vi "Main.vi"(11 "Error In":errorcluster) -> (15 "Error Out":errorcluster)   [LabVIEW 2020]
doc: "The VI is a launcher VI that allows to perform the sender to receiver communication"
uses:
  Controls/Queue Operation.ctl
  Controls/User Event Operations.ctl
  Controls/Launcher Data.ctl
  Classes/Sender/Methods/Sender UI.vi
  Classes/Sender/Sender.lvclass
  Classes/Receiver/Methods/Receiver UI.vi
  Classes/Receiver/Receiver.lvclass
panel:
  # "Instructions:\n1. Run the VI.\n2. View the sender and receiver loaded in the front panel.\n3. Select the transmission data type.\n4. Click the notify button to send notification to the receiver.\n5. Click notify with data to send one data at a time.\n6. Click stream data to continuously stream data to the receiver and click stop stream to stop.\n7. Click panel close to stop the VI running"
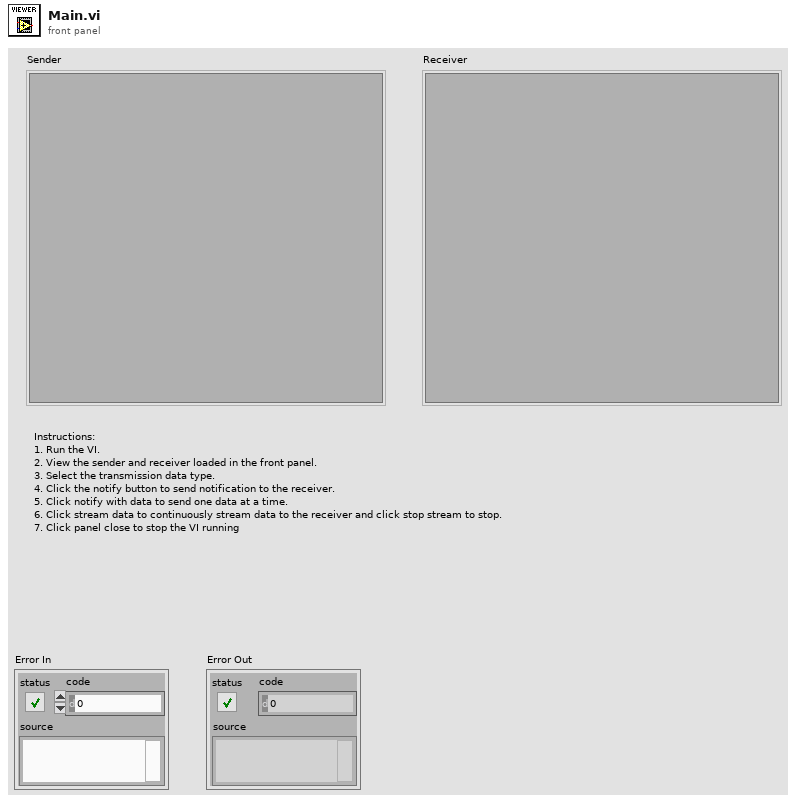
[diagram p1: front panel]
types:
  T1 = typedef "Launcher Data.ctl" = cluster{"Sender Reference":refnum<vi>, "Receiver Reference":refnum<vi>}
  T2 = typedef "User Event Operations.ctl" = enum16{"Obtain", "Generate", "Destroy"}
  T3 = typedef "Queue Operation.ctl" = enum16{"Create & Enqueue N", "Enqueue N", "Dequeue", "Enstack N", "Flush", "Release"}
  T4 = typedef "Queue Element.ctl" = cluster{"State":string, "Data":variant}
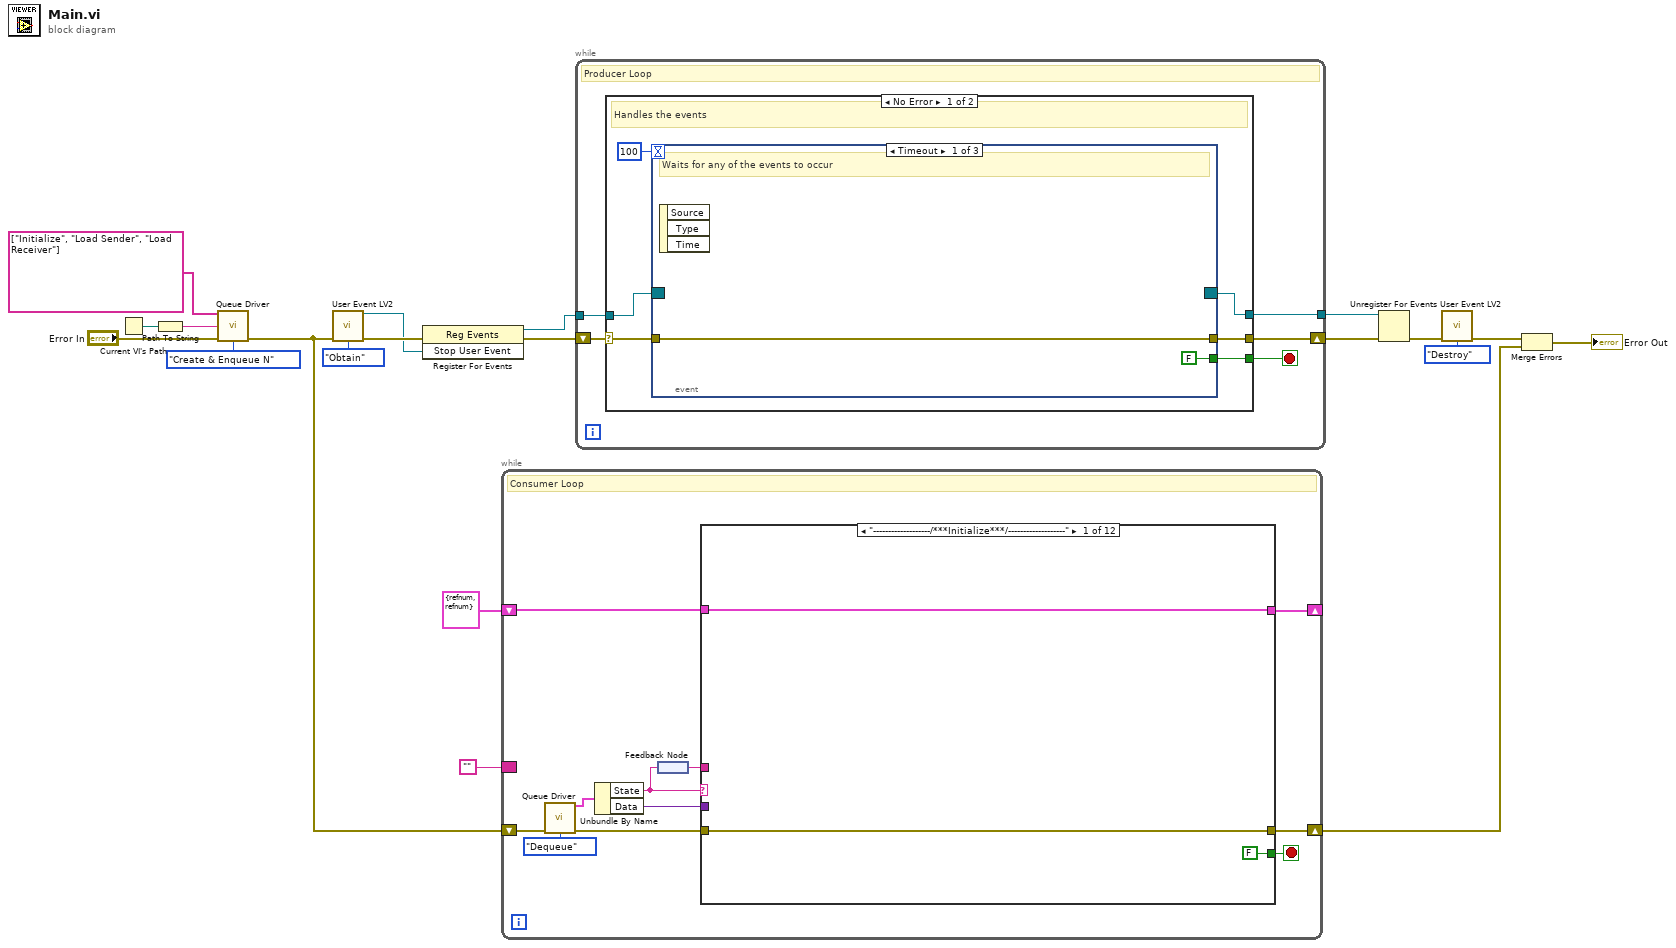
[diagram p0: block diagram]
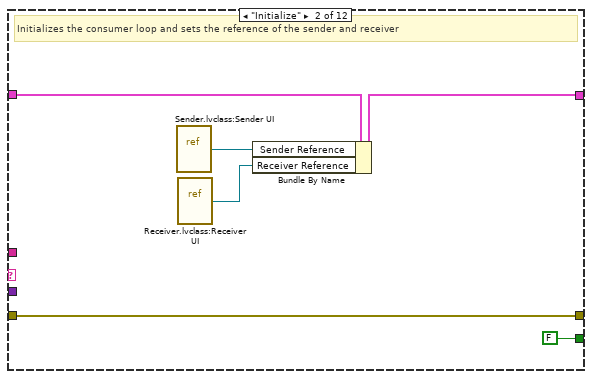
[diagram p2: hidden frame]
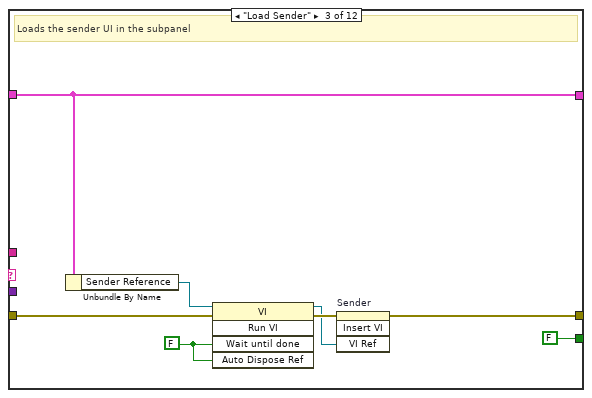
[diagram p3: hidden frame]
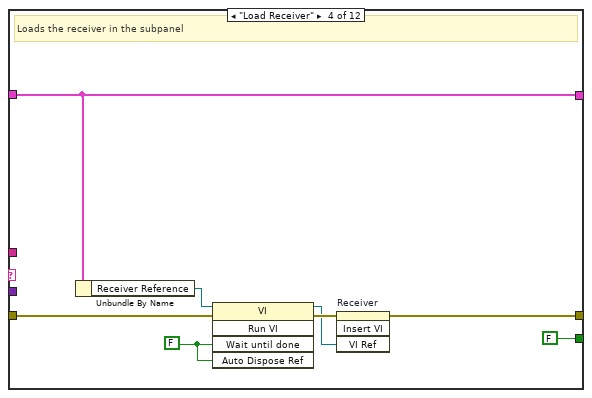
[diagram p4: hidden frame]
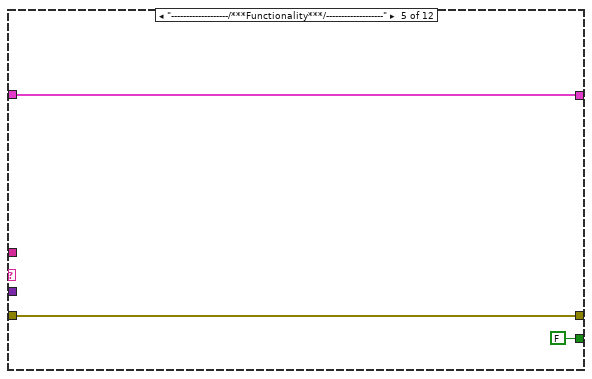
[diagram p5: hidden frame]
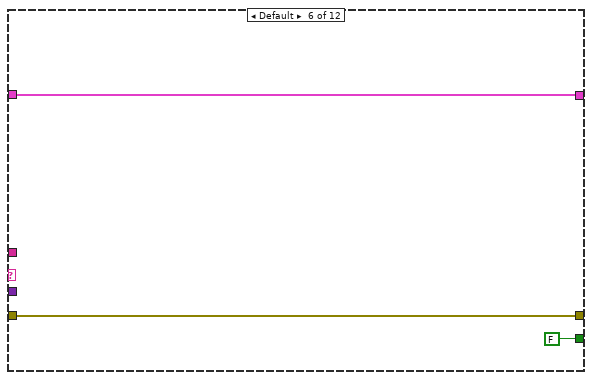
[diagram p6: hidden frame]
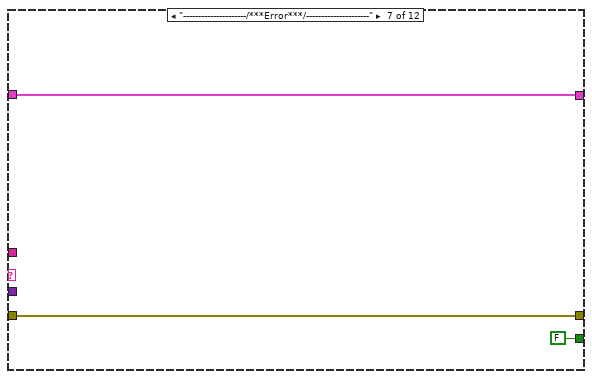
[diagram p7: hidden frame]
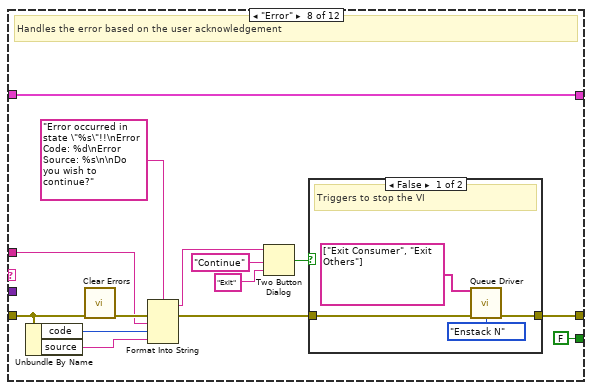
[diagram p8: hidden frame]
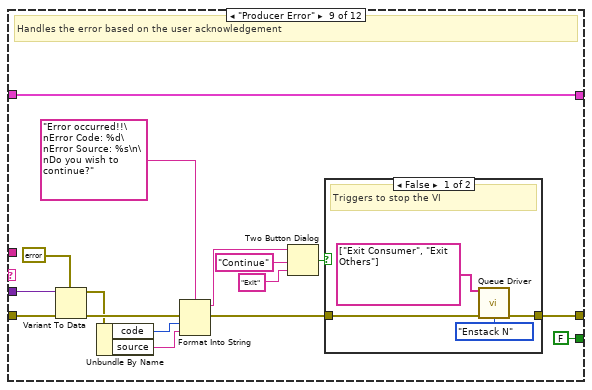
[diagram p10: hidden frame]
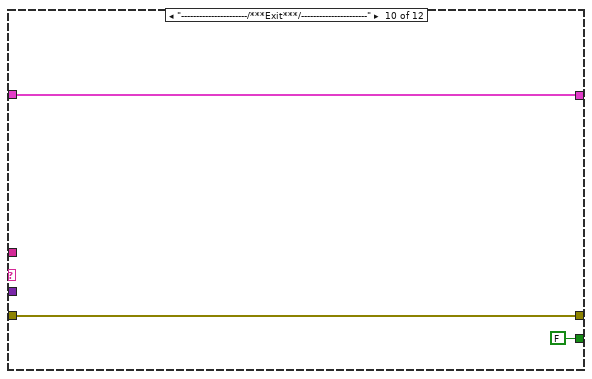
[diagram p12: hidden frame]
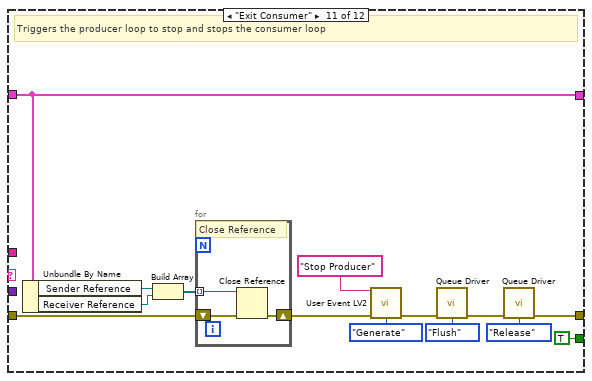
[diagram p13: hidden frame]
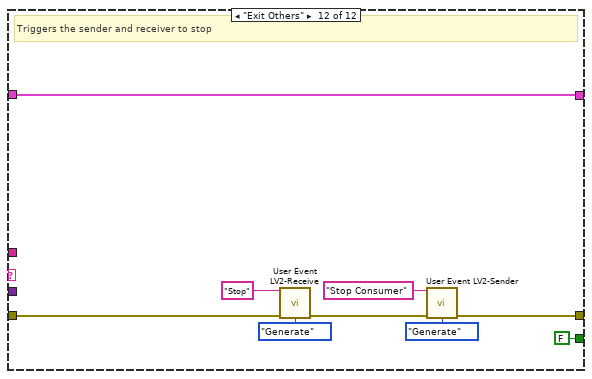
[diagram p14: hidden frame]
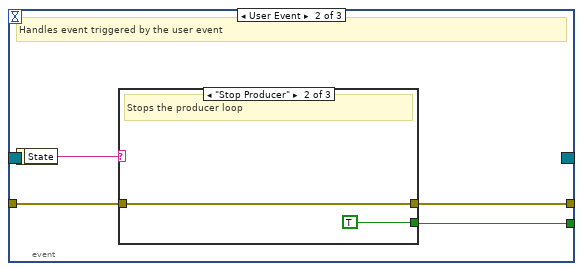
[diagram p15: hidden frame]
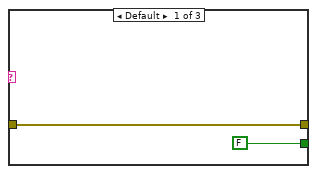
[diagram p16: hidden frame]
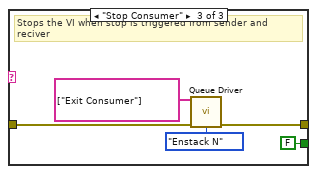
[diagram p17: hidden frame]
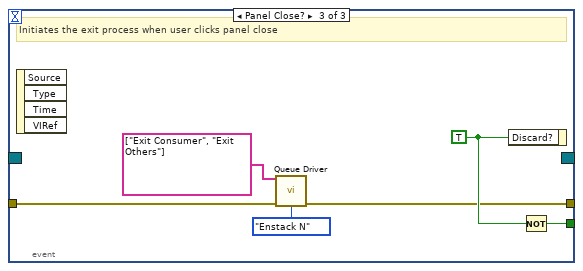
[diagram p18: hidden frame]
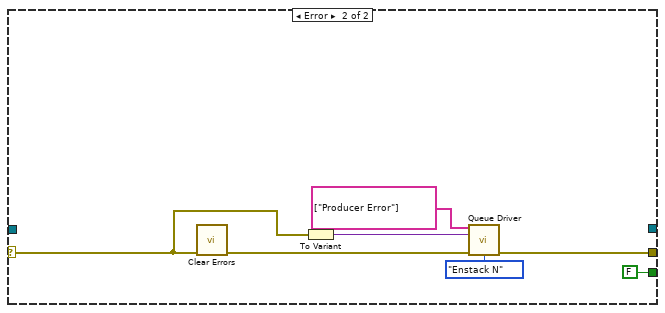
[diagram p19: hidden frame]
diagram:
  n1 = Current VI's Path() -> (path=w17:path)
  n2 = Path To String(path=w17) -> (string=w1:string)
  n3 = call "Queue Driver.vi"("States[]"=string[] ["Initialize", "Load Sender", "Load Receiver"], "Queue Name"=w1, "Error In"="Error In", "Queue Operation"=Queue_Operation."Create & Enqueue N") -> ("Error Out"=w11:errorcluster)  [unwired: 10 in, 1 out]
  n4 = call "User Event LV2.vi"("Error In"=w11, "Operation"=User_Event_Operations."Obtain") -> ("Stop User Event"=w9:refnum<user-event>, "Error Out"=w13:errorcluster)  [unwired: 12 in]
  n5 = register-events(error in=w13, w9) -> (reference out=w8:refnum<event-registration>, error out=w10:errorcluster)  [unwired: 1 in]
  n6 = while {
    shift-right: [w30] -> w14
    shift-left: w11 -> [w31]
    border: "" -> [_]
    shift-right: [w23] -> _
    shift-left: T1 {"Sender Reference"=refnum, "Receiver Reference"=refnum} -> [w24]
    stop <- w27 stop-if-true
    # "Consumer Loop"
    n7 = call "Queue Driver.vi"("Error In"=w31, "Queue Operation"=Queue_Operation."Dequeue") -> ("Dequeue Element"=w21:T4, "Error Out"=w29:errorcluster)  [unwired: 12 in]
    n8 = Unbundle By Name(w21) -> ("State"=w26:string, "Data"=w22:variant)
    n9 = feedback-in #1(w26) -> ()
    n10 = feedback #1() -> (w25:string)
    n11 = case shown="\"-------------------/***Initialize***/-------------------\"" w26 {
      tunnel: w29 -> [w34 w35 w48 w56 w59 w62 w65 w71 w95 w108 w122 w134]
      tunnel: [w34 w35 w45 w53 w59 w62 w65 w68 w93 w108 w118 w128] -> w30
      tunnel: [FALSE FALSE FALSE FALSE FALSE FALSE FALSE FALSE FALSE FALSE TRUE FALSE] -> w27
      tunnel: w25 -> [_ _ _ _ _ _ _ w69 _ _ _ _]
      tunnel: w24 -> [w32 w39 w42 w50 w57 w60 w63 w66 w91 w106 w112 w132]
      tunnel: [w32 w38 w42 w50 w57 w60 w63 w66 w91 w106 w112 w132] -> w23
      tunnel: w22 -> [_ _ _ _ _ _ _ _ w90 _ _ _]
      frame "-------------------/***Initialize***/-------------------" {
      }
      frame "Initialize" {
        # "Initializes the consumer loop and sets the reference of the sender and receiver"
        n12 = vi-ref "Sender.lvclass:Sender UI.vi"() -> (w37:refnum<vi>)
        n13 = vi-ref "Receiver.lvclass:Receiver UI.vi"() -> (w36:refnum<vi>)
        n14 = Bundle By Name(cluster=w39, "Sender Reference"=w37, "Receiver Reference"=w36) -> (w38:T1)
      }
      frame "Load Sender" {
        w43 = FALSE ("Wait Until Done")
        # "Loads the sender UI in the subpanel"
        n15 = Unbundle By Name(w42) -> ("Sender Reference"=w41:refnum<vi>)
        n16 = invoke class="VI" method="Run VI"(reference=w41, error in=w48, "Wait until done"=w43, "Auto Dispose Ref"=w43) -> (reference out=w44:refnum<vi>, error out=w46:errorcluster)  [unwired: 1 in, 3 out]
        n17 = invoke on="Sender" class="SubPnl" method="Insert VI"(error in=w46, "VI Ref"=w44) -> (error out=w45:errorcluster)  [unwired: 2 in, 3 out]
      }
      frame "Load Receiver" {
        w51 = FALSE ("Wait Until Done")
        # "Loads the receiver in the subpanel"
        n18 = Unbundle By Name(w50) -> ("Receiver Reference"=w49:refnum<vi>)
        n19 = invoke class="VI" method="Run VI"(reference=w49, error in=w56, "Wait until done"=w51, "Auto Dispose Ref"=w51) -> (reference out=w52:refnum<vi>, error out=w54:errorcluster)  [unwired: 1 in, 3 out]
        n20 = invoke on="Receiver" class="SubPnl" method="Insert VI"(error in=w54, "VI Ref"=w52) -> (error out=w53:errorcluster)  [unwired: 2 in, 3 out]
      }
      frame "-------------------/***Functionality***/-------------------" {
      }
      frame Default {
      }
      frame "---------------------/***Error***/---------------------" {
      }
      frame "Error" {
        # "Handles the error based on the user acknowledgement"
        n21 = Unbundle By Name(w71) -> ("code"=w73:i32, "source"=w72:string)
        n22 = call <vilib>:"Clear Errors.vi"("error in (no error)"=w71) -> ("error out"=w78:errorcluster)  [unwired: 5 in, 1 out]
        n23 = Format Into String(format string="Error occurred in state \"%s\"!!\nError Code: %d\nError Source: %s\n\nDo you wish to continue?", error in=w78, w69, w73, w72) -> (resulting string=w76:string, error out=w70:errorcluster)  [unwired: 1 in]
        n24 = Two Button Dialog(message=w76, 1:"Exit" ("F button name (\"Cancel\")"), 2:"Continue" ("T button name (\"OK\")")) -> (T button?=w67:bool)
        n25 = case shown="False" w67 {
          tunnel: w70 -> [w83 w84]
          tunnel: [w82 w84] -> w68
          frame False {
            # "Triggers to stop the VI"
            n26 = call "Queue Driver.vi"("States[]"=string[] ["Exit Consumer", "Exit Others"], "Error In"=w83, "Queue Operation"=Queue_Operation."Enstack N") -> ("Error Out"=w82:errorcluster)  [unwired: 11 in, 1 out]
          }
          frame True {
          }
        }
      }
      frame "Producer Error" {
        # "Handles the error based on the user acknowledgement"
        n27 = Variant To Data(error in=w95, type=errorcluster {"status"=FALSE, "code"=0, "source"=""} ("error out"), Variant=w90) -> (data=w87:errorcluster, error out=w89:errorcluster)
        n28 = Unbundle By Name(w87) -> ("code"=w86:i32, "source"=w85:string)
        n29 = Format Into String(format string="Error occurred!!\nError Code: %d\nError Source: %s\n\nDo you wish to continue?", error in=w89, w86, w85) -> (resulting string=w98:string, error out=w94:errorcluster)  [unwired: 1 in]
        n30 = Two Button Dialog(message=w98, 1:"Exit" ("F button name (\"Cancel\")"), 2:"Continue" ("T button name (\"OK\")")) -> (T button?=w92:bool)
        n31 = case shown="False" w92 {
          tunnel: w94 -> [w104 w105]
          tunnel: [w103 w105] -> w93
          frame False {
            # "Triggers to stop the VI"
            n32 = call "Queue Driver.vi"("States[]"=string[] ["Exit Consumer", "Exit Others"], "Error In"=w104, "Queue Operation"=Queue_Operation."Enstack N") -> ("Error Out"=w103:errorcluster)  [unwired: 11 in, 1 out]
          }
          frame True {
          }
        }
      }
      frame "----------------------/***Exit***/----------------------" {
      }
      frame "Exit Consumer" {
        # "Triggers the producer loop to stop and stops the consumer loop"
        n33 = Unbundle By Name(w112) -> ("Sender Reference"=w111:refnum<vi>, "Receiver Reference"=w110:refnum<vi>)
        n34 = Build Array(w111, w110) -> (w109:refnum<vi>[])
        n35 = for {
          shift-right: [w124] -> w113
          shift-left: w122 -> [w125]
          tunnel: w109 -> [w123] mode=indexing
          # "Close Reference"
          n36 = Close Reference(reference=w123, error in (no error)=w125) -> (error out=w124:errorcluster)
        }
        n37 = call "User Event LV2.vi"("Event Name"="Stop Producer", "Error In"=w113, "Operation"=User_Event_Operations."Generate") -> ("Error Out"=w116:errorcluster)  [unwired: 11 in, 1 out]
        n38 = call "Queue Driver.vi"("Error In"=w116, "Queue Operation"=Queue_Operation."Flush") -> ("Error Out"=w120:errorcluster)  [unwired: 12 in, 1 out]
        n39 = call "Queue Driver.vi"("Error In"=w120, "Queue Operation"=Queue_Operation."Release") -> ("Error Out"=w118:errorcluster)  [unwired: 12 in, 1 out]
      }
      frame "Exit Others" {
        # "Triggers the sender and receiver to stop"
        n40 = call "User Event LV2-Receive.vi"("Event Name"="Stop", "Error In"=w134, "Operation"=User_Event_Operations."Generate") -> ("Error Out"=w131:errorcluster)  [unwired: 11 in, 1 out]
        n41 = call "User Event LV2-Sender.vi"("Event Name"="Stop Consumer", "Error In"=w131, "Operation"=User_Event_Operations."Generate") -> ("Error Out"=w128:errorcluster)  [unwired: 11 in, 1 out]
      }
    }
  }
  n42 = while {
    shift-right: [w137] -> w19
    shift-left: w10 -> [w138]
    tunnel: w8 -> [w136]
    tunnel: [w135] -> w6
    stop <- w139 stop-if-true
    # "Producer Loop"
    n43 = case shown="No Error" w138 {
      selector: w138 -> [w144 w168]
      tunnel: [w145 FALSE] -> w139
      tunnel: [w143 w171] -> w137
      tunnel: w136 -> [w141 _]
      tunnel: [w140 _] -> w135
      frame No Error {
        # "Handles the events"
        n44 = event shown="[0] Timeout" {
          selector: w141 -> [_ _ _]
          dyn-events: [_ _ _] -> w140
          timeout: 100 -> [_ _ _]
          tunnel: [FALSE w148 w165] -> w145
          tunnel: w144 -> [w146 w151 w164]
          tunnel: [w146 w150 w163] -> w143
          event Timeout {
            # "Waits for any of the events to occur"
            n45 = event-data() -> ()  [unwired: 1 in, 3 out]
          }
          event User Event {
            # "Handles event triggered by the user event"
            n46 = event-data() -> ("State"=w149:string)  [unwired: 1 in]
            n47 = case shown="\"Stop Producer\"" w149 {
              tunnel: w151 -> [w153 w155 w160]
              tunnel: [w153 w155 w158] -> w150
              tunnel: [FALSE TRUE FALSE] -> w148
              frame Default {
              }
              frame "Stop Producer" {
                # "Stops the producer loop"
              }
              frame "Stop Consumer" {
                # "Stops the VI when stop is triggered from sender and reciver"
                n48 = call "Queue Driver.vi"("States[]"=string[] ["Exit Consumer"], "Error In"=w160, "Queue Operation"=Queue_Operation."Enstack N") -> ("Error Out"=w158:errorcluster)  [unwired: 11 in, 1 out]
              }
            }
          }
          event Panel Close? {
            w166 = TRUE ("Discard?")
            # "Initiates the exit process when user clicks panel close"
            n49 = event-data() -> ()  [unwired: 1 in, 4 out]
            n50 = call "Queue Driver.vi"("States[]"=string[] ["Exit Consumer", "Exit Others"], "Error In"=w164, "Queue Operation"=Queue_Operation."Enstack N") -> ("Error Out"=w163:errorcluster)  [unwired: 11 in, 1 out]
            n51 = event-data("Discard?"=w166) -> ()  [unwired: 1 in, 1 out]
            n52 = Not(x=w166) -> (.not. x?=w165:bool)
          }
        }
      }
      frame Error {
        n53 = call <vilib>:"Clear Errors.vi"("error in (no error)"=w168) -> ("error out"=w172:errorcluster)  [unwired: 5 in, 1 out]
        n54 = To Variant(anything=w168) -> (Variant=w167:variant)
        n55 = call "Queue Driver.vi"("States[]"=string[] ["Producer Error"], "Data"=w167, "Error In"=w172, "Queue Operation"=Queue_Operation."Enstack N") -> ("Error Out"=w171:errorcluster)  [unwired: 10 in, 1 out]
      }
    }
  }
  n56 = Unregister For Events(event registration refnum=w6, error in=w19) -> (error out=w7:errorcluster)
  n57 = call "User Event LV2.vi"("Error In"=w7, "Operation"=User_Event_Operations."Destroy") -> ("Error Out"=w5:errorcluster)  [unwired: 12 in, 1 out]
  n58 = Merge Errors(w5, w14) -> (→"Error Out":errorcluster)
